vi "DPIDs.vi"(8 "error in (no error)":errorcluster, 11 "Node Ptr":T1 format="%.0x") -> (0 "error out":errorcluster)   [LabVIEW 2019, in "Diagnostics Addon System Explorer.lvlib"]
uses:
  Diagnostics Addon System Explorer.lvlib
  <vilib>/NI VeriStand/Custom Device API/Custom Device Item Ref.ctl
  Types/FG.Action.ctl
  SubVIs/ID.FG.vi
  Addon Shared/SubVIs/Constants.vi
  <vilib>/NI VeriStand/Custom Device Tools/Custom Device Utility Library/NI VeriStand - Search for All Items by GUID.vi
  <vilib>/NI/NI VeriStand Advanced SysDef API/SysDef API/SysDef.Property.Set.vi
  <vilib>/NI/NI VeriStand Advanced SysDef API/_SubVIs/SysDef.Property.Set.U32.vi
  <vilib>/NI VeriStand/Custom Device API/NI VeriStand - Get Item Property.vi
  <vilib>/NI VeriStand/Custom Device API/Get Item Property (U32).vi
  <vilib>/NI/NI VeriStand Advanced SysDef API/_SubVIs/SysDef.Property.Set.U32.Array.vi
  <vilib>/NI VeriStand/Custom Device API/Get Item Property (U32 Array).vi
  <vilib>/NI VeriStand/Custom Device API/Custom Device API.lvlib
  <vilib>/NI VeriStand/Custom Device Tools/Custom Device Utility Library/Custom Device Utility Library.lvlib
  Addon Shared/Diagnostics Addon Shared.lvlib
panel:
  in  "SHDocVw.IWebBrowser":refnum<k7>(container)
  out "DPIDs":i32(listbox)
  in  "Description":string
  out "Name":string
  in  "Header":cluster{"Section Name":string}={"Section Name"="Custom Device Item Settings"}
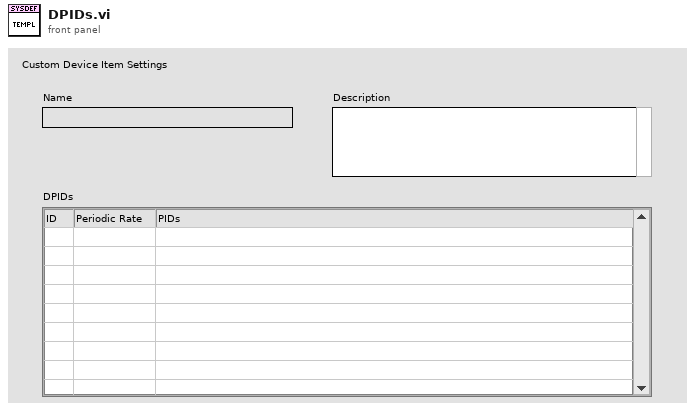
[diagram p1: front panel]
types:
  T1 = typedef "Custom Device API.lvlib/Custom Device Item Ref.ctl" = u64
  T2 = typedef "Diagnostics Addon System Explorer.lvlib/FG.Action.ctl" = enum16{"Get", "Set"}
  T3 = typedef "Custom Device API.lvlib/Custom Device Item Info.ctl" = cluster{"Name":string, "Is Channel":bool, "GUID":string, "Is Waveform":bool}
  T4 = typedef "Diagnostics Addon Shared.lvlib/DPID.ctl" = cluster{"DPID ID":u8, "Speed":T5, "PIDs":u16[]}
  T5 = typedef "Diagnostics Addon Shared.lvlib/DPID.Rate.ctl" = enum16{"Slow", "Medium", "Fast"}
  T6 = typedef "Custom Device API.lvlib/Custom Device Commands.ctl" = enum16{"Default", "Item renamed", "Shutdown", "Dynamic button pressed"}
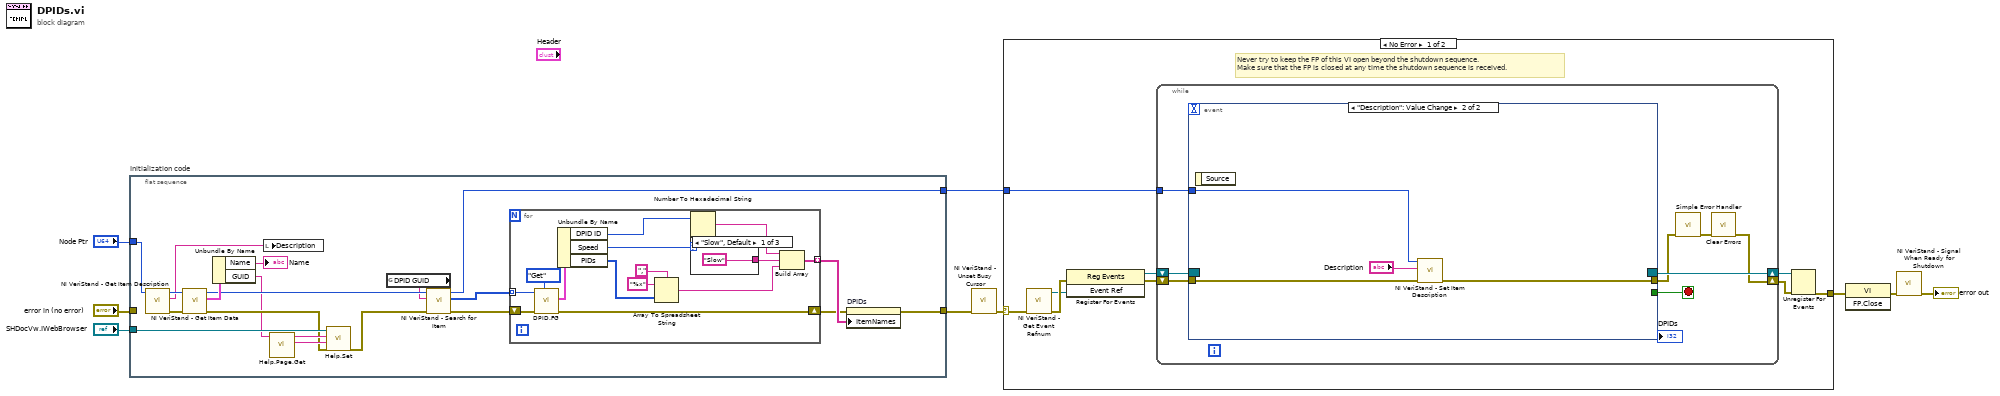
[diagram p0: block diagram]
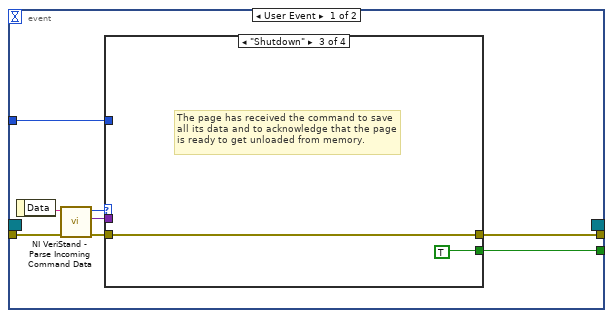
[diagram p2: hidden frame]
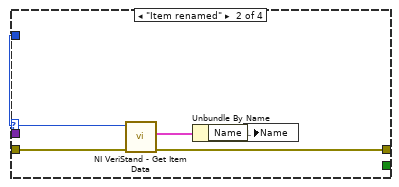
[diagram p4: hidden frame]
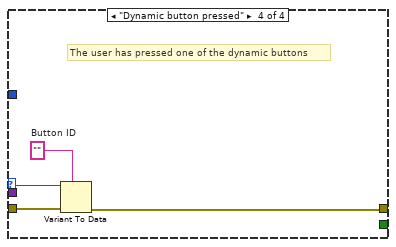
[diagram p5: hidden frame]
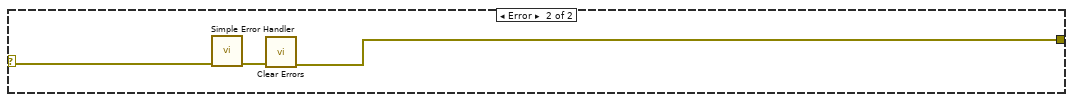
[diagram p6: hidden frame]
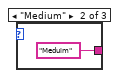
[diagram p7: hidden frame]
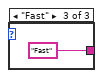
[diagram p8: hidden frame]
diagram:
  n1 = flat-sequence "Initialization code" {
    tunnel: "error in (no error)" -> [_]
    tunnel: "Node Ptr" -> [w28]
    tunnel: [w17] -> w5
    tunnel: [w22] -> w2
    tunnel: "SHDocVw.IWebBrowser" -> [w24]
    frame #0 {
      n2 = call <vilib>:"NI VeriStand - Get Item Description.vi"("Item Ref in"=w28) -> ("error out"=w26:errorcluster, "Description"=w27:string, "Item Ref out"=w29:T1)  [unwired: 1 in, 7 out]
      n3 = call <vilib>:"NI VeriStand - Get Item Data.vi"("error in (no error)"=w26, "Item Ref in"=w29) -> ("error out"=w13:errorcluster, "Item Info"=w25:T3, "Item Ref out"=w23:T1)  [unwired: 7 out]
      n4 = Unbundle By Name(w25) -> ("Name"=→"Name":string, "GUID"=w11:string)
      n5 = local write "Description"(w27) -> ()
      n6 = call "Help.Page.Get.vi"("GUID"=w11) -> ("HTML File"=w15:string, "Main CHM File"=w14:string)  [unwired: 9 in]
      n7 = call "Help.Set.vi"("error in (no error)"=w13, "HTML File"=w15, "Main CHM File"=w14, "SHDocVw.IWebBrowser2"=w24) -> ("error out"=w12:errorcluster)  [unwired: 7 in]
      n8 = global read "Constants.vi" "DPID GUID"() -> (w10:string)
      n9 = call-poly <vilib>:"NI VeriStand - Search for Item.vi"("error in"=w12, "Item GUID"=w10, "Section Ref in"=w23) -> ("error out"=w20:errorcluster, "Item Refs"=w21:T1[], "Section Ref out"=w22:T1)  [unwired: 5 in, 1 out]
      n10 = for {
        tunnel: w21 -> [w43] mode=indexing
        shift-right: [w41] -> w18
        shift-left: w20 -> [w42]
        tunnel: [w31] -> w19 mode=indexing
        n11 = call "DPID.FG.vi"("Action"=FG.Action."Get", "error in (no error)"=w42, "Device Item Ref in"=w43) -> ("error out"=w41:errorcluster, "DPID"=w40:T4)  [unwired: 6 in, 1 out]
        n12 = Unbundle By Name(w40) -> ("DPID ID"=w39:u8, "Speed"=w38:T5, "PIDs"=w37:u16[])
        n13 = Array To Spreadsheet String(delimiter (Tab)=",", array=w37, 3:"%x" ("format string")) -> (spreadsheet string=w32:string)
        n14 = Number To Hexadecimal String(2:w39) -> (0:w34:string)  [unwired: 1 in]
        n15 = case shown="\"Slow\", Default" w38 {
          tunnel: ["Slow" "Meduim" "Fast"] -> w33
          frame "Slow", Default {
          }
          frame "Medium" {
          }
          frame "Fast" {
          }
        }
        n16 = Build Array(w34, w33, w32) -> (w31:string[])
      }
      n17 = property on="DPIDs" class="MCListbox (strict)"(error in=w18, "ItemNames"=w19) -> (error out=w17:errorcluster)  [unwired: 1 in, 1 out]
    }
  }
  n18 = call <vilib>:"NI VeriStand - Unset Busy Cursor.vi"("error in (no error)"=w5) -> ("error out"=w4:errorcluster)  [unwired: 10 out]
  n19 = case shown="No Error" w4 {
    selector: w4 -> [w47 w90]
    tunnel: [w52 w88] -> w9
    tunnel: w2 -> [w48 _]
    frame No Error {
      # "Never try to keep the FP of this VI open beyond the shutdown sequence.\nMake sure that the FP is closed at any time the shutdown sequence is received."
      n20 = call <vilib>:"NI VeriStand - Get Event Refnum.vi"("error in (no error)"=w47) -> ("error out"=w55:errorcluster, "Event Ref"=w51:refnum<user-event>)  [unwired: 9 out]
      n21 = register-events(error in=w55, w51) -> (reference out=w49:refnum<event-registration>, error out=w50:errorcluster)  [unwired: 1 in]
      n22 = while {
        tunnel: w48 -> [w59]
        shift-right: [w56] -> w53
        shift-left: w50 -> [w62]
        shift-right: [w63] -> w54
        shift-left: w49 -> [w61]
        stop <- w60 stop-if-true
        n23 = event shown="[1] \"Description\": Value Change" {
          selector: w61 -> [_ _]
          dyn-events: [_ _] -> w63
          timeout: _ -> [_ _]
          tunnel: w62 -> [w71 w86]
          tunnel: [w67 _] -> w60
          tunnel: [w66 w85] -> w58
          tunnel: w59 -> [w65 w87]
          event User Event {
            n24 = event-data() -> ("Data"=w70:string)  [unwired: 1 out]
            n25 = call <vilib>:"NI VeriStand - Parse Incoming Command Data.vi"("error in (no error)"=w71, "Incoming data"=w70) -> ("error out"=w69:errorcluster, "Outgoing data"=w64:variant, "Action"=w68:T6)  [unwired: 7 out]
            n26 = case shown="\"Shutdown\"" w68 {
              tunnel: w69 -> [w72 w77 w78 w83]
              tunnel: [_ _ TRUE _] -> w67
              tunnel: [w72 w74 w78 w80] -> w66
              tunnel: w65 -> [_ w76 _ _]
              tunnel: w64 -> [_ _ _ w82]
              frame "Default", Default {
              }
              frame "Item renamed" {
                n27 = call <vilib>:"NI VeriStand - Get Item Data.vi"("error in (no error)"=w77, "Item Ref in"=w76) -> ("error out"=w74:errorcluster, "Item Info"=w75:T3)  [unwired: 8 out]
                n28 = Unbundle By Name(w75) -> ("Name"=w73:string)
                n29 = local write "Name"(w73) -> ()
              }
              frame "Shutdown" {
                # "The page has received the command to save all its data and to acknowledge that the page is ready to get unloaded from memory."
              }
              frame "Dynamic button pressed" {
                w81 = ""  # Button ID
                # "The user has pressed one of the dynamic buttons"
                n30 = Variant To Data(error in=w83, type=w81, Variant=w82) -> (error out=w80:errorcluster)  [unwired: 1 out]
              }
            }
          }
          event "Description": Value Change {
            n31 = event-data() -> ()  [unwired: 2 out]
            n32 = call <vilib>:"NI VeriStand - Set Item Description.vi"("error in (no error)"=w86, "Description"="Description", "Item Ref in"=w87) -> ("error out"=w85:errorcluster)  [unwired: 8 out]
          }
        }
        n33 = call <vilib>:"Simple Error Handler.vi"("error in (no error)"=w58) -> ("error out"=w57:errorcluster)  [unwired: 1 in, 7 out]
        n34 = call <vilib>:"Clear Errors.vi"("error in (no error)"=w57) -> ("error out"=w56:errorcluster)  [unwired: 1 in, 5 out]
      }
      n35 = Unregister For Events(event registration refnum=w54, error in=w53) -> (error out=w52:errorcluster)
    }
    frame Error {
      n36 = call <vilib>:"Simple Error Handler.vi"("error in (no error)"=w90) -> ("error out"=w89:errorcluster)  [unwired: 1 in, 7 out]
      n37 = call <vilib>:"Clear Errors.vi"("error in (no error)"=w89) -> ("error out"=w88:errorcluster)  [unwired: 1 in, 5 out]
    }
  }
  n38 = invoke class="VI" method="FP.Close"(error in=w9) -> (error out=w8:errorcluster)  [unwired: 2 in, 2 out]
  n39 = call <vilib>:"NI VeriStand - Signal When Ready for Shutdown.vi"("error in (no error)"=w8) -> ("error out"=→"error out":errorcluster)  [unwired: 10 out]
